vi "rqcBob Set Initial Seed for Ramdom Number Generator.vi"(8 "error in":errorcluster, 10 "rndGen.initial seed":u32, 11 "FPGA reference in":refnum<k20>) -> (0 "error out":errorcluster, 3 "FPGA reference out":refnum<k20>)   [LabVIEW 2016]
uses:
  <vilib>/Utility/error.llb/Error Cluster From Error Code.vi
  <vilib>/rvi/errors/niLvFpgaAdjustHostInterfaceError.vi
  <vilib>/rvi/interface/nirviReadWriteControl/nirviReadWriteControl.xnode
  NiFpgaLv.dll
  <vilib>/rvi/interface/Simulation/niFpgaSimulationCallBeginRW.vi
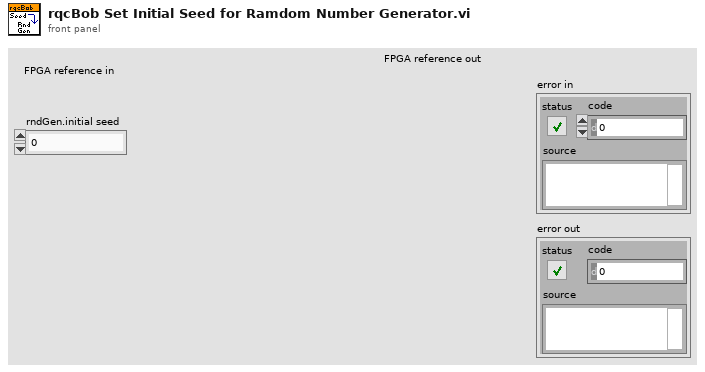
[diagram p1: front panel]
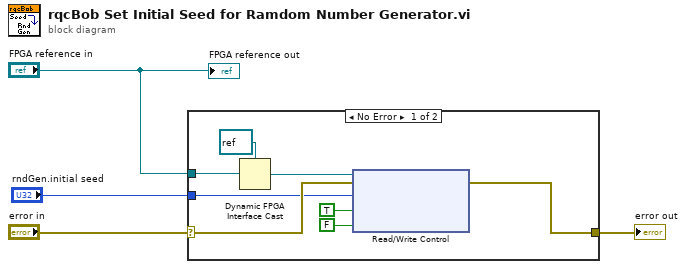
[diagram p0: block diagram]
diagram:
  n1 = case shown="No Error" "error in" {
    selector: "error in" -> [w12 w13]
    tunnel: [w11 w13] -> w2
    tunnel: "FPGA reference in" -> [w9 _]
    tunnel: "rndGen.initial seed" -> [w5 _]
    frame No Error {
      n2 = Dynamic FPGA Interface Cast(Session In=refnum<k20> refnum ("FPGA Interface"), Type=w9) -> (Session Out=w8:refnum<k20>)
      n3 = xnode "Read/Write Control"("FPGA VI Reference In"=w8, "error in"=w12, "rndGen.initial seed"=w5, "rndGen.reset"=TRUE, "rndGen.reset"=FALSE) -> ("error out"=w11:errorcluster)  [unwired: 1 out]
    }
    frame Error {
    }
  }
  "error out" <- w2
  "FPGA reference out" <- "FPGA reference in"
